vi "DSF.Shared.Configuration.Channel.Get Type.vi"(11 "Channel Configuration in":refnum<class "DSF.Shared.Configuration.Channel.lvclass">) -> (2 "data type":T1, 3 "Channel Configuration out":refnum<class "DSF.Shared.Configuration.Channel.lvclass">)   [LabVIEW 2017, in "DSF.Engine.lvlib" / "DSF.Shared.Configuration.Channel.lvclass"]
uses:
  DSF.Shared.Configuration.Channel.lvclass
  DSF Configuration API/1.0.0/Public/Controls/DSF Data Type.ctl
  DSF.Shared.Configuration.Channel.lvclass/DSF.Shared.Configuration.Channel.ctl
  DSF Configuration API/1.0.0/DSF Configuration API.lvlib
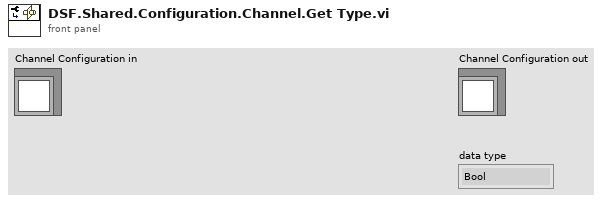
[diagram p1: front panel]
types:
  T1 = typedef "DSF Configuration API.lvlib/DSF Data Type.ctl" = enum8{"Bool", "SGL", "DBL", "I8", "I16", "I32", "I64", "U8", "U16", "U32", "U64"}
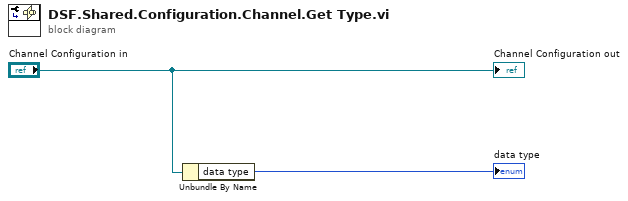
[diagram p0: block diagram]
diagram:
  n1 = Unbundle By Name("Channel Configuration in") -> ("data type"=→"data type":T1)
  "Channel Configuration out" <- "Channel Configuration in"
